vi "Receiver_Example - 2 Channel - Experiment_5.vi"() -> ()   [LabVIEW 2022 SP3]
panel:
  in  "Channel":bool
  in  "Tab Control 2":enum32{"1 Channel", "2 Channel"}(tab)
  out "Constellation Map 1 Channel":cdb[](graph)
  out "Low-Power BER - 1 Channel":dbl(graph)
  out "High-Power BER - 1 Channel":dbl(graph)
  out "High-Power Decoded message - 1 Channel":string
  out "Low-Power Decoded message - 1 Channel":string
  out "Low-Power Decoded message - CH0":string
  out "Decoded message - CH1":string
  out "Constellation Map 2 Channel":cluster{"Constellation":cdb[]}[](graph)
  out "Low-Power BER - CH0":dbl(graph)
  out "High-Power BER":T1(graph)
  out "High-Power Decoded message - CH0":string
  out "CH1 2":bool
  out "CH0 2":bool
  in  "Counter":dbl
  in  "State":i32
  out "iterationsIM":dbl
  out "High-Power Image 2":T2(plugin-control)
  in  "High-Power Window Size":dbl=15.0 format="%#_6p"
  in  "Low-Power Window Size - CH0":dbl=15.0 format="%#_6p"
  in  "Tab Control":enum32{"USRP Parameters", "Rx Info", "BER"}(tab)
  in  "USRP ControledParameters":T3={"Active Antenna"="RX2", "Gain (dB)"=10.0, "Carrier Frequency"=2400000000.0, "IQ Rate"=2000000.0, "Active channels"="0,1"} {"IQ Rate" format="%#_6p"; "Carrier Frequency" format="%#_6p"; "Gain (dB)" format="%#_6f"}
  in  "Device selection":refnum<k15>="RIO0"
  in  "Trigger level":dbl=0.005 format="%f"
  out "CH0":T4
  out "CH1":T4
  out "SIG valid? - CH1":bool
  out "SIG valid? - CH0":bool
  out "Frequency offset - CH1":dbl
  out "Frequency offset - CH0":dbl
  out "Coerced Parameters":T5={"IQ Rate"=100000.0, "Carrier  Freq."=100000.0, "Gain"=0.0} {"Gain" format="%#_6f"; "Carrier  Freq." format="%#_6p"; "IQ Rate" format="%#_6p"}
  out "Error out":errorcluster
  in  "Expected message LP - CH0":string="Non Critical Data\nNon Critical Data\nNon Critical Data\nNon Critical Data\nNon Critical Data"
  in  "Expected message - CH1":string="Critical Dataaaaa\nCritical Dataaaaa\nCritical Dataaaaa\nCritical Dataaaaa\nCritical Dataaaaa"
  out "Expected message LP Detected CH0":string="Non Critical Data\nNon Critical Data\nNon Critical Data\nNon Critical Data\nNon Critical Data"
  out "Expected message HP Detected CH1":string="Non Critical Data\nNon Critical Data\nNon Critical Data\nNon Critical Data\nNon Critical Data"
  in  "Boolean":bool
  in  "Boolean 3":bool
  out "Expected message HP Detected CH0":string="Non Critical Data\nNon Critical Data\nNon Critical Data\nNon Critical Data\nNon Critical Data"
  in  "Expected message HP - CH0":string="Critical Dataaaaa\nCritical Dataaaaa\nCritical Dataaaaa\nCritical Dataaaaa\nCritical Dataaaaa"
  in  "Boolean 2":bool
  out "Inst. BER HP - CH0":dbl format="%#_4g"
  out "Acc. BER HP - CH0":dbl format="%#_4g"
  out "Acum. Err HP - CH0":dbl
  out "No. Bits HP - CH0":dbl
  out "Acc. BER LP - CH0":dbl format="%#_4g"
  out "Inst. BER - CH1":dbl format="%#_4g"
  out "Inst. BER LP - CH0":dbl format="%#_4g"
  out "No. Bits - CH1":dbl
  out "No. Bits LP - CH0":dbl
  out "Acum. Err - CH1":dbl
  out "Acum. Err LP - CH0":dbl
  in  "Record BER":bool
  in  "Refresh Button":bool
  out "Acc. BER - CH1":dbl format="%#_4g"
  in  "error in (no error)":errorcluster
  # "OFDM Superposition Coded Receiver"
  # "1 Channel"
  # "2 Channel"
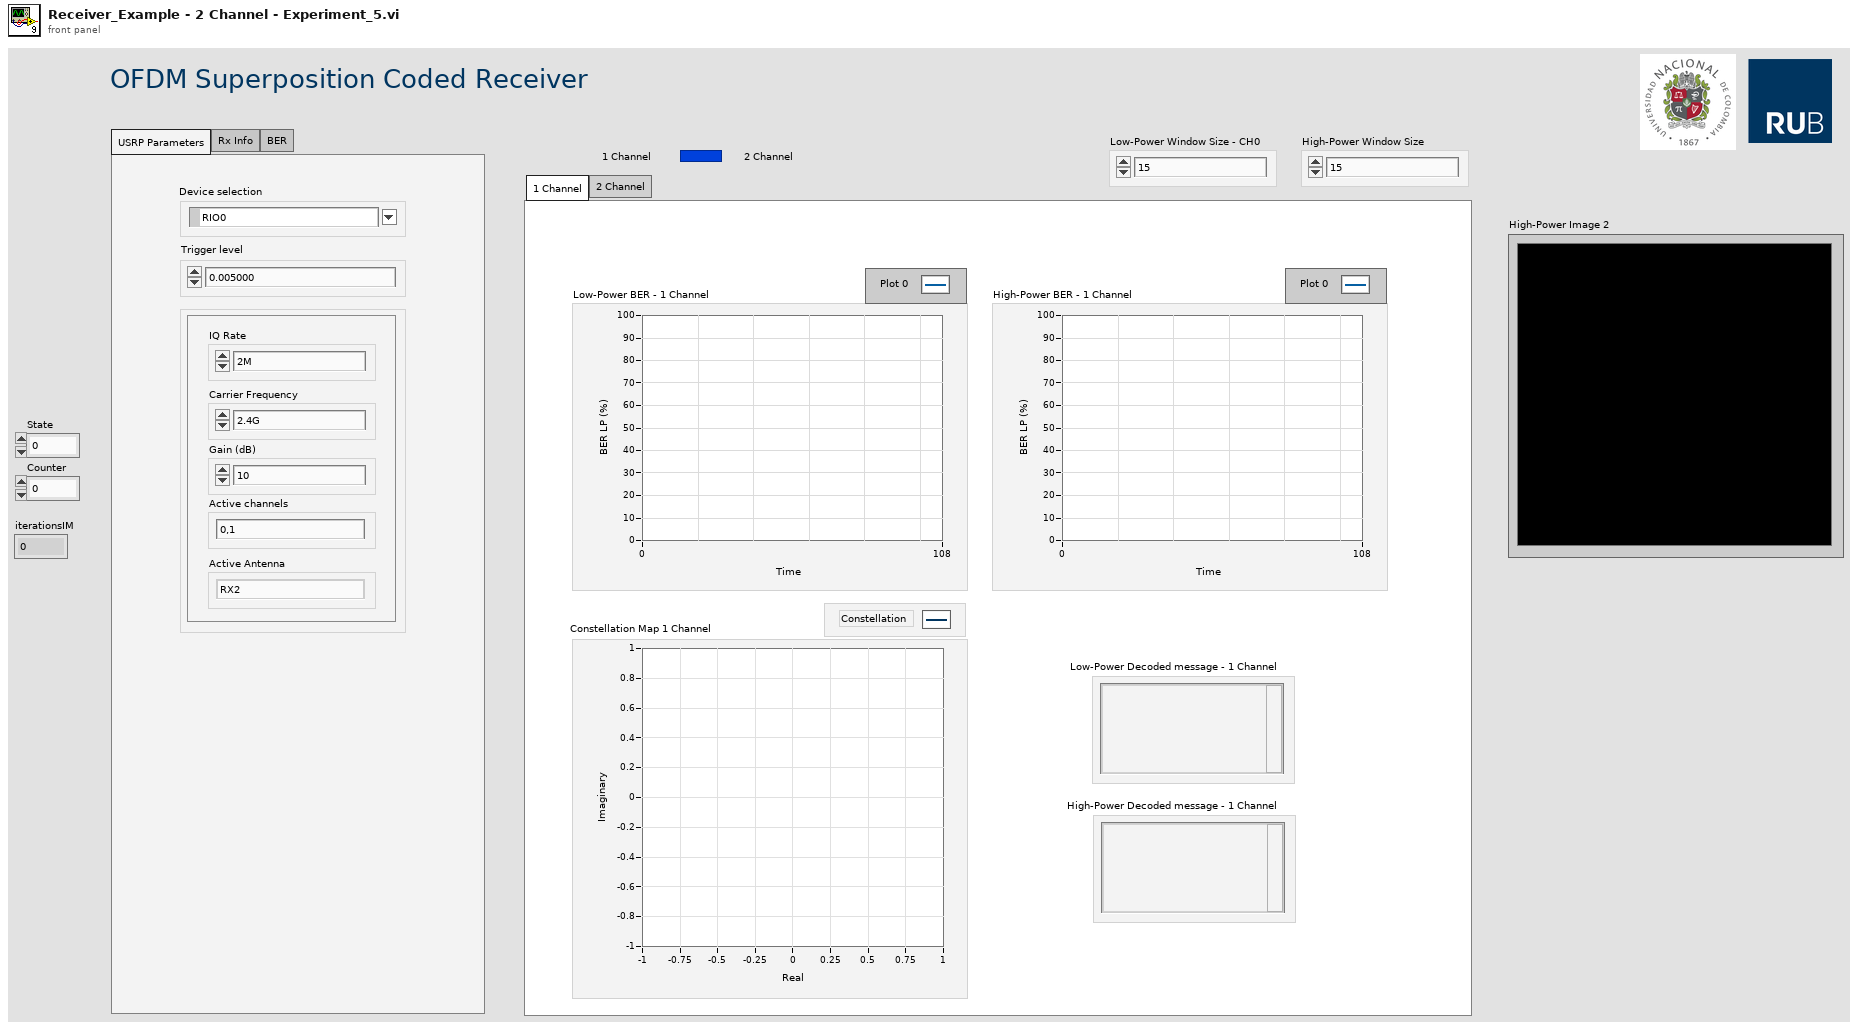
[diagram p1: front panel]
types:
  T1 = cluster{"Graph Instantaneous BER":dbl, "Graph Instantaneous BER":dbl, "Inst. BER - CH1":dbl}
  T2 = typedef "IMAQ Image.ctl" = refnum<image>
  T3 = cluster{"Active Antenna":string, "Gain (dB)":dbl, "Carrier Frequency":dbl, "IQ Rate":dbl, "Active channels":string}
  T4 = cluster{"Modulation type":enum16{"QPSK(4QAM)", "64QAM", "16QAM", "BPSK"}, "BCC rate (k/n)":enum16{"1/2", "2/3", "3/4"}}
  T5 = cluster{"IQ Rate":dbl, "Carrier  Freq.":dbl, "Gain":dbl}
  T6 = cluster{"coerced IQ rate":dbl, "coerced carrier frequency":dbl, "coerced gain":dbl}
  T7 = cluster{"Graph Instantaneous BER":dbl, "Graph Instantaneous BER":dbl, "Graph Instantaneous BER":dbl}
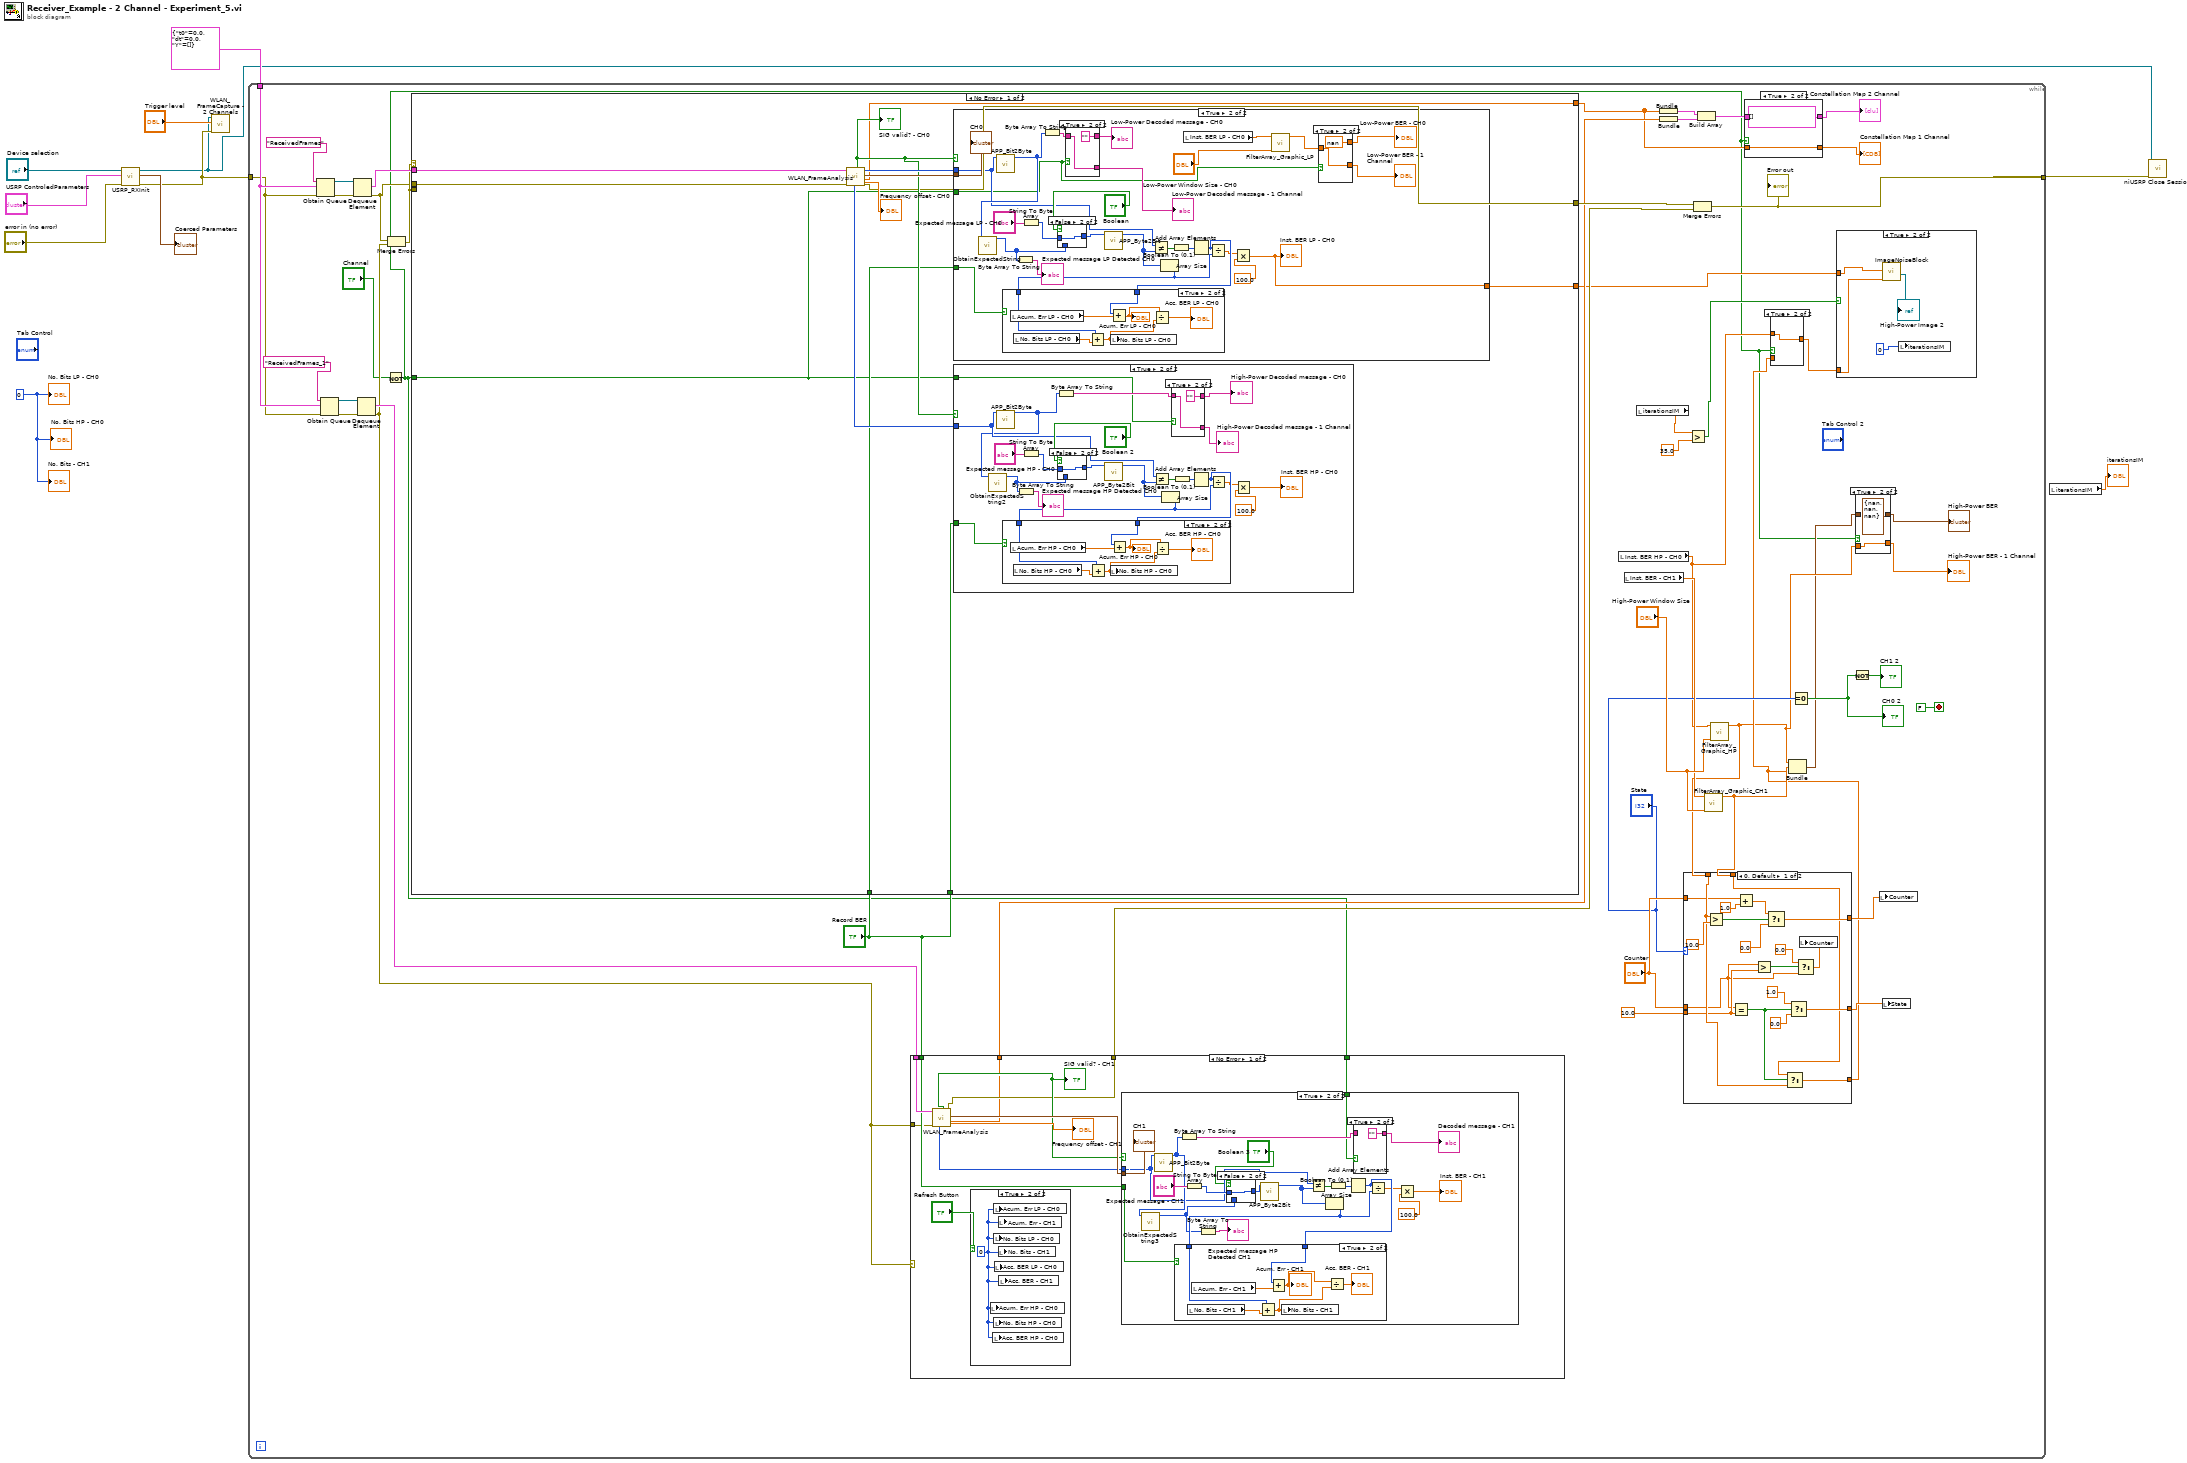
[diagram p0: block diagram]
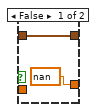
[diagram p2: hidden frame]
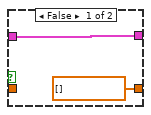
[diagram p4: hidden frame]
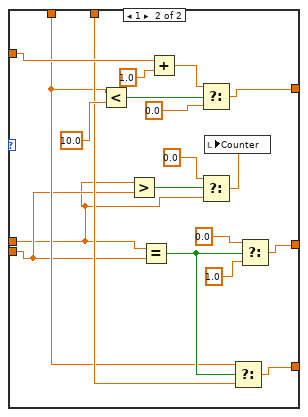
[diagram p5: hidden frame]
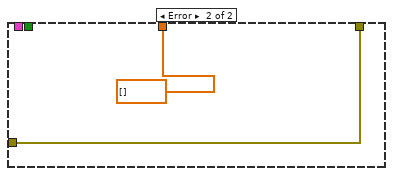
[diagram p11: hidden frame]
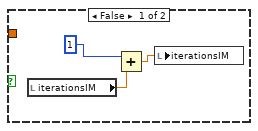
[diagram p12: hidden frame]
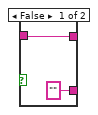
[diagram p14: hidden frame]
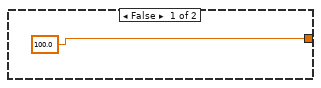
[diagram p17: hidden frame]
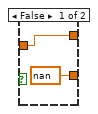
[diagram p18: hidden frame]
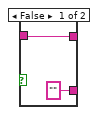
[diagram p19: hidden frame]
diagram:
  w2 = 0
  n1 = call "USRP_RXInit.vi"("device names"="Device selection", "USRP ControledParameters"="USRP ControledParameters", "error in (no error)"="error in (no error)") -> ("session handle out"=w5:refnum<k15>, "USRP CoercedParamters"=→"Coerced Parameters":T6, "error out"=w9:errorcluster)  [unwired: 5 in]
  n2 = call "WLAN_FrameCapture - 2 Channels.vi"("error in (no error)"=w9, "Trigger level"="Trigger level", "session handle"=w5) -> ()  [unwired: 8 in]
  n3 = while {
    tunnel: w9 -> [w51]
    tunnel: cluster{"t0":dbl, "dt":dbl, "Y":cdb[]} {"t0"=0.0, "dt"=0.0, "Y"=[]} ("data") -> [w52]
    tunnel: [w40] -> w6
    stop <- FALSE stop-if-true
    n4 = Obtain Queue(name (unnamed)="ReceivedFrames", element data type=w52, error in (no error)=w51) -> (queue out=w59:refnum<queue>, error out=w57:errorcluster)  [unwired: 2 in, 1 out]
    n5 = Obtain Queue(name (unnamed)="ReceivedFrames_1", element data type=w52, error in (no error)=w51) -> (queue out=w55:refnum<queue>, error out=w54:errorcluster)  [unwired: 2 in, 1 out]
    n6 = Dequeue Element(queue=w59, error in (no error)=w57) -> (element=w58:cluster{"t0":dbl, "dt":dbl, "Y":cdb[]}, error out=w48:errorcluster)  [unwired: 1 in, 2 out]
    n7 = Dequeue Element(queue=w55, error in (no error)=w54) -> (element=w43:cluster{"t0":dbl, "dt":dbl, "Y":cdb[]}, error out=w38:errorcluster)  [unwired: 1 in, 2 out]
    n8 = Not(x="Channel") -> (.not. x?=w12:bool)
    n9 = Merge Errors(w48, w38) -> (w49:errorcluster)
    n10 = case shown="No Error" w49 {
      tunnel: w58 -> [w170 _]
      tunnel: w49 -> [_ w254]
      tunnel: w48 -> [w167 _]
      tunnel: [w166 100] -> w36
      tunnel: [w165 dbl[] []] -> w24
      tunnel: [w164 w254] -> w42
      tunnel: "Record BER" -> [w163 _]
      tunnel: "Record BER" -> [w162 _]
      tunnel: w12 -> [w161 _]
      frame No Error {
        n11 = call "WLAN_FrameAnalysis.vi"("error in (no error)"=w167, "input cluster"=w170) -> ("error out"=w164:errorcluster, "Constellation"=w165:cdb[], "Modulation parameter"=w171:T4, "output bits"=w172:i8[], "Frequency offset"=→"Frequency offset - CH0":dbl, "SIG valid?"=w168:bool, "outputbitsHP"=w169:i8[])  [unwired: 3 in]
        "SIG valid? - CH0" <- w168
        n12 = case shown="True" w168 {
          tunnel: w172 -> [_ w217]
          tunnel: w171 -> [_ w235]
          tunnel: w162 -> [_ w231]
          tunnel: [100.0 w216] -> w166
          tunnel: w161 -> [_ w209]
          frame False {
          }
          frame True {
            n13 = call "APP_Bit2Byte.vi"("input bit stream"=w217) -> ("output byte stream"=w221:u8[])  [unwired: 10 in]
            n14 = call "ObtainExpectedString.vi"("Array"=w221) -> ("detectedMessage"=w218:i8[])  [unwired: 9 in]
            n15 = Byte Array To String(unsigned byte array=w218) -> (string=→"Expected message LP Detected CH0":string)
            n16 = String To Byte Array(string="Expected message LP - CH0") -> (unsigned byte array=w222:u8[])
            n17 = Byte Array To String(unsigned byte array=w221) -> (string=w215:string)
            n18 = case shown="False" "Boolean" {
              tunnel: [w244 w245] -> w224
              tunnel: w222 -> [_ w245]
              tunnel: w218 -> [w244 _]
              frame True {
              }
              frame False {
              }
            }
            n19 = case shown="True" w209 {
              tunnel: w215 -> [w241 w243]
              tunnel: ["" ("string") w243] -> w214
              tunnel: [w241 "" ("string")] -> w213
              frame False {
              }
              frame True {
              }
            }
            "Low-Power Decoded message - CH0" <- w213
            "Low-Power Decoded message - 1 Channel" <- w214
            n20 = call "APP_Byte2Bit.vi"("input byte stream"=w224) -> ("output bit stream"=w223:i8[])  [unwired: 10 in]
            n21 = Not Equal?(x=w217, y=w223) -> (x != y?=w233:bool[])
            n22 = Array Size(array=w223) -> (size(s)=w230:i32)
            n23 = Boolean To (0,1)(Boolean=w233) -> (0, 1=w234:i16[])
            n24 = local read "Inst. BER LP - CH0"() -> (w227:dbl)
            n25 = Add Array Elements(numeric array=w234) -> (sum=w229:i16)
            n26 = case shown="True" w231 {
              tunnel: w230 -> [_ w251]
              tunnel: w229 -> [_ w249]
              frame False {
              }
              frame True {
                n27 = local read "Acum. Err LP - CH0"() -> (w250:dbl)
                n28 = local read "No. Bits LP - CH0"() -> (w252:dbl)
                n29 = Add(x=w251, y=w252) -> (x+y=w248:dbl)
                n30 = Add(x=w249, y=w250) -> (x+y=w247:dbl)
                "Acum. Err LP - CH0" <- w247
                n31 = local write "No. Bits LP - CH0"(w248) -> ()
                n32 = Divide(x=w247, y=w248) -> (x/y=→"Acc. BER LP - CH0":dbl)
              }
            }
            n33 = Divide(x=w229, y=w230) -> (x/y=w226:dbl)
            n34 = Multiply(x=w226, y=100.0) -> (x*y=w216:dbl)
            "Inst. BER LP - CH0" <- w216
            n35 = call "FilterArray_Graphic_LP.vi"("Window Size"="Low-Power Window Size - CH0", "Instantaneous BER"=w227) -> ("Graph Instantaneous BER"=w212:dbl)  [unwired: 4 in, 1 out]
            n36 = case shown="True" w209 {
              tunnel: w212 -> [w237 w239]
              tunnel: [nan ("Graph Instantaneous BER") w239] -> w211
              tunnel: [w237 nan ("Graph Instantaneous BER")] -> w210
              frame False {
              }
              frame True {
              }
            }
            "Low-Power BER - CH0" <- w210
            "Low-Power BER - 1 Channel" <- w211
            "CH0" <- w235
          }
        }
        n37 = case shown="True" w168 {
          tunnel: w169 -> [_ w181]
          tunnel: w163 -> [_ w191]
          tunnel: w161 -> [_ w174]
          frame False {
          }
          frame True {
            n38 = call "APP_Bit2Byte.vi"("input bit stream"=w181) -> ("output byte stream"=w180:u8[])  [unwired: 10 in]
            n39 = call "ObtainExpectedString2.vi"("Array"=w180) -> ("detectedMessage"=w179:i8[])  [unwired: 9 in]
            n40 = Byte Array To String(unsigned byte array=w179) -> (string=→"Expected message HP Detected CH0":string)
            n41 = String To Byte Array(string="Expected message HP - CH0") -> (unsigned byte array=w184:u8[])
            n42 = Byte Array To String(unsigned byte array=w180) -> (string=w175:string)
            n43 = case shown="False" "Boolean 2" {
              tunnel: [w199 w200] -> w186
              tunnel: w184 -> [_ w200]
              tunnel: w179 -> [w199 _]
              frame True {
              }
              frame False {
              }
            }
            n44 = call "APP_Byte2Bit.vi"("input byte stream"=w186) -> ("output bit stream"=w185:i8[])  [unwired: 10 in]
            n45 = Not Equal?(x=w181, y=w185) -> (x != y?=w193:bool[])
            n46 = Array Size(array=w185) -> (size(s)=w190:i32)
            n47 = case shown="True" w174 {
              tunnel: w175 -> [w196 w198]
              tunnel: ["" ("string") w198] -> w176
              tunnel: [w196 "" ("string")] -> w177
              frame False {
              }
              frame True {
              }
            }
            "High-Power Decoded message - CH0" <- w177
            "High-Power Decoded message - 1 Channel" <- w176
            n48 = Boolean To (0,1)(Boolean=w193) -> (0, 1=w194:i16[])
            n49 = Add Array Elements(numeric array=w194) -> (sum=w189:i16)
            n50 = case shown="True" w191 {
              tunnel: w190 -> [_ w206]
              tunnel: w189 -> [_ w204]
              frame False {
              }
              frame True {
                n51 = local read "Acum. Err HP - CH0"() -> (w205:dbl)
                n52 = local read "No. Bits HP - CH0"() -> (w207:dbl)
                n53 = Add(x=w206, y=w207) -> (x+y=w203:dbl)
                n54 = local write "No. Bits HP - CH0"(w203) -> ()
                n55 = Add(x=w204, y=w205) -> (x+y=w202:dbl)
                "Acum. Err HP - CH0" <- w202
                n56 = Divide(x=w202, y=w203) -> (x/y=→"Acc. BER HP - CH0":dbl)
              }
            }
            n57 = Divide(x=w189, y=w190) -> (x/y=w188:dbl)
            n58 = Multiply(x=w188, y=100.0) -> (x*y=→"Inst. BER HP - CH0":dbl)
          }
        }
      }
      frame Error {
        (unwired) 100
      }
    }
    n59 = case shown="No Error" w38 {
      tunnel: w43 -> [w114 _]
      tunnel: "Record BER" -> [w112 _]
      tunnel: [w111 w153] -> w41
      tunnel: [w110 dbl[] []] -> w39
      tunnel: w38 -> [w109 w153]
      tunnel: w12 -> [w108 _]
      frame No Error {
        n60 = call "WLAN_FrameAnalysis.vi"("error in (no error)"=w109, "input cluster"=w114) -> ("error out"=w111:errorcluster, "Constellation"=w110:cdb[], "Modulation parameter"=w117:T4, "Frequency offset"=→"Frequency offset - CH1":dbl, "SIG valid?"=w113:bool, "outputbitsHP"=w115:i8[])  [unwired: 3 in, 1 out]
        "SIG valid? - CH1" <- w113
        n61 = case shown="True" "Refresh Button" {
          frame False {
          }
          frame True {
            w119 = 0
            n62 = local write "Acum. Err HP - CH0"(w119) -> ()
            n63 = local write "Acc. BER HP - CH0"(w119) -> ()
            n64 = local write "Acum. Err LP - CH0"(w119) -> ()
            n65 = local write "No. Bits LP - CH0"(w119) -> ()
            n66 = local write "No. Bits HP - CH0"(w119) -> ()
            n67 = local write "Acc. BER LP - CH0"(w119) -> ()
            n68 = local write "Acum. Err - CH1"(w119) -> ()
            n69 = local write "No. Bits - CH1"(w119) -> ()
            n70 = local write "Acc. BER - CH1"(w119) -> ()
          }
        }
        n71 = case shown="True" w113 {
          tunnel: w115 -> [_ w126]
          tunnel: w117 -> [_ w140]
          tunnel: w112 -> [_ w123]
          tunnel: w108 -> [_ w120]
          frame False {
          }
          frame True {
            n72 = call "APP_Bit2Byte.vi"("input bit stream"=w126) -> ("output byte stream"=w129:u8[])  [unwired: 10 in]
            n73 = call "ObtainExpectedString3.vi"("Array"=w129) -> ("detectedMessage"=w128:i8[])  [unwired: 9 in]
            n74 = Byte Array To String(unsigned byte array=w129) -> (string=w121:string)
            n75 = String To Byte Array(string="Expected message - CH1") -> (unsigned byte array=w130:u8[])
            n76 = Byte Array To String(unsigned byte array=w128) -> (string=→"Expected message HP Detected CH1":string)
            n77 = case shown="False" "Boolean 3" {
              tunnel: [w143 w144] -> w132
              tunnel: w130 -> [_ w144]
              tunnel: w128 -> [w143 _]
              frame True {
              }
              frame False {
              }
            }
            n78 = call "APP_Byte2Bit.vi"("input byte stream"=w132) -> ("output bit stream"=w131:i8[])  [unwired: 10 in]
            n79 = Not Equal?(x=w126, y=w131) -> (x != y?=w138:bool[])
            n80 = Array Size(array=w131) -> (size(s)=w136:i32)
            n81 = Boolean To (0,1)(Boolean=w138) -> (0, 1=w139:i16[])
            n82 = Add Array Elements(numeric array=w139) -> (sum=w135:i16)
            n83 = case shown="True" w123 {
              tunnel: w136 -> [_ w150]
              tunnel: w135 -> [_ w148]
              frame False {
              }
              frame True {
                n84 = local read "No. Bits - CH1"() -> (w151:dbl)
                n85 = local read "Acum. Err - CH1"() -> (w149:dbl)
                n86 = Add(x=w150, y=w151) -> (x+y=w147:dbl)
                n87 = Add(x=w148, y=w149) -> (x+y=w146:dbl)
                "Acum. Err - CH1" <- w146
                n88 = local write "No. Bits - CH1"(w147) -> ()
                n89 = Divide(x=w146, y=w147) -> (x/y=→"Acc. BER - CH1":dbl)
              }
            }
            n90 = case shown="True" w120 {
              tunnel: w121 -> [w141 _]
              tunnel: [w141 "" ("string")] -> w122
              frame False {
              }
              frame True {
              }
            }
            "Decoded message - CH1" <- w122
            n91 = Divide(x=w135, y=w136) -> (x/y=w133:dbl)
            n92 = Multiply(x=w133, y=100.0) -> (x*y=→"Inst. BER - CH1":dbl)
            "CH1" <- w140
          }
        }
      }
      frame Error {
      }
    }
    n93 = local read "Inst. BER HP - CH0"() -> (w19:dbl)
    n94 = local read "Inst. BER - CH1"() -> (w30:dbl)
    n95 = local read "iterationsIM"() -> (w47:dbl)
    n96 = Bundle("Constellation"=w24) -> (w25:cluster{"Constellation":cdb[]})  [unwired: 1 in]
    n97 = Bundle("Constellation"=w39) -> (w44:cluster{"Constellation":cdb[]})  [unwired: 1 in]
    n98 = Greater?(x=w47, y=35.0) -> (0:w46:bool)
    n99 = Merge Errors(w42, w41) -> (w40:errorcluster)
    "Error out" <- w40
    n100 = Build Array(w25, w44) -> (w22:cluster{"Constellation":cdb[]}[])
    n101 = call "FilterArray_Graphic_CH1.vi"("Window Size"="High-Power Window Size", "Instantaneous BER"=w30) -> ("Graph Instantaneous BER"=w29:dbl)  [unwired: 4 in, 1 out]
    n102 = call "FilterArray_Graphic_HP.vi"("Window Size"="High-Power Window Size", "Instantaneous BER"=w19) -> ("Graph Instantaneous BER"=w16:dbl)  [unwired: 4 in, 1 out]
    n103 = case shown="0, Default" "State" {
      tunnel: "Counter" -> [w76 w96]
      tunnel: [w83 w99] -> w34
      tunnel: "Counter" -> [w71 w89]
      tunnel: [w80 w98] -> w33
      tunnel: [w78 w97] -> w17
      tunnel: w16 -> [w77 w94]
      tunnel: w29 -> [w75 w95]
      tunnel: 10.0 ("y") -> [w74 w90]
      frame 0, Default {
        n104 = Greater?(x=w77, y=10.0) -> (0:w84:bool)
        n105 = Equal?(x=w71, y=w74) -> (x = y?=w79:bool)
        n106 = Add(x=w76, y=1.0) -> (x+y=w86:dbl)
        n107 = Greater?(x=w71, y=w74) -> (0:w73:bool)
        n108 = Select(t=w86, s=w84, f=0.0) -> (s? t:f=w83:dbl)
        n109 = Select(t=w75, s=w79, f=w77) -> (s? t:f=w78:dbl)
        n110 = Select(t=1.0, s=w79, f=0.0) -> (s? t:f=w80:dbl)
        n111 = Select(t=0.0, s=w73, f=w71) -> (s? t:f=w70:dbl)
        n112 = local write "Counter"(w70) -> ()
      }
      frame 1 {
        n113 = Less?(x=w94, y=10.0) -> (x < y?=w100:bool)
        n114 = Greater?(x=w89, y=w90) -> (0:w92:bool)
        n115 = Equal?(x=w89, y=w90) -> (x = y?=w102:bool)
        n116 = Add(x=w96, y=1.0) -> (x+y=w106:dbl)
        n117 = Select(t=w106, s=w100, f=0.0) -> (s? t:f=w99:dbl)
        n118 = Select(t=0.0, s=w92, f=w89) -> (s? t:f=w93:dbl)
        n119 = local write "Counter"(w93) -> ()
        n120 = Select(t=w94, s=w102, f=w95) -> (s? t:f=w97:dbl)
        n121 = Select(t=0.0, s=w102, f=1.0) -> (s? t:f=w98:dbl)
      }
    }
    n122 = case shown="True" w12 {
      tunnel: [cdb[] [] ("Constellation") w69] -> w23
      tunnel: w24 -> [_ w69]
      tunnel: w22 -> [w67 _]
      tunnel: [w67 cluster{"Constellation":cdb[]}[] []] -> w21
      frame False {
      }
      frame True {
      }
    }
    "Constellation Map 2 Channel" <- w21
    "Constellation Map 1 Channel" <- w23
    n123 = case shown="True" w12 {
      tunnel: w19 -> [_ w65]
      tunnel: [w64 w65] -> w18
      tunnel: w17 -> [w64 _]
      frame False {
      }
      frame True {
      }
    }
    n124 = Bundle("Graph Instantaneous BER"=w16, "Graph Instantaneous BER"=w29, "Graph Instantaneous BER"=w17) -> (w14:T7)  [unwired: 1 in]
    n125 = Equal To 0?(x="State") -> (x = 0?=w26:bool)
    "CH0 2" <- w26
    n126 = case shown="True" w46 {
      tunnel: w18 -> [_ w160]
      tunnel: w36 -> [_ w157]
      frame False {
        n127 = local read "iterationsIM"() -> (w156:dbl)
        n128 = Add(x=1, y=w156) -> (x+y=w155:dbl)
        n129 = local write "iterationsIM"(w155) -> ()
      }
      frame True {
        n130 = call "ImageNoiseBlock.vi"("BERLP"=w157, "BERHP"=w160) -> ("High-Power Image"=→"High-Power Image 2":T2)  [unwired: 8 in]
        n131 = local write "iterationsIM"(0) -> ()
      }
    }
    n132 = Not(x=w26) -> (.not. x?=→"CH1 2":bool)
    n133 = case shown="True" w12 {
      tunnel: w16 -> [_ w63]
      tunnel: [nan w63] -> w15
      tunnel: w14 -> [w61 _]
      tunnel: [w61 T7 {"Graph Instantaneous BER"=nan, "Graph Instantaneous BER"=nan, "Graph Instantaneous BER"=nan}] -> w13
      frame False {
      }
      frame True {
      }
    }
    "High-Power BER" <- w13
    "High-Power BER - 1 Channel" <- w15
    n134 = local write "Counter"(w34) -> ()
    n135 = local write "State"(w33) -> ()
  }
  n136 = local read "iterationsIM"() -> (→"iterationsIM":dbl)
  n137 = call <instrlib>:"niUSRP Close Session.vi"("session handle"=w5, "error in (no error)"=w6) -> ()  [unwired: 13 in, 1 out]
  "No. Bits LP - CH0" <- w2
  "No. Bits - CH1" <- w2
  "No. Bits HP - CH0" <- w2
